vi "writeToXML.vi"(8 "error in (no error)":errorcluster, 10 "classLabel":string, 11 "StartUp in":refnum<class "StartUp.lvclass">) -> (0 "error out":errorcluster, 2 "XML out":string, 3 "StartUp out":refnum<class "StartUp.lvclass">)   [LabVIEW 2022 SP3, in "TCSDataDefinitions.lvlib" / "TCSCommand.lvlib" / "StartUp.lvclass"]
uses:
  StartUp.lvclass
  TCSTcsCommand/TCSTcsCommand.lvclass
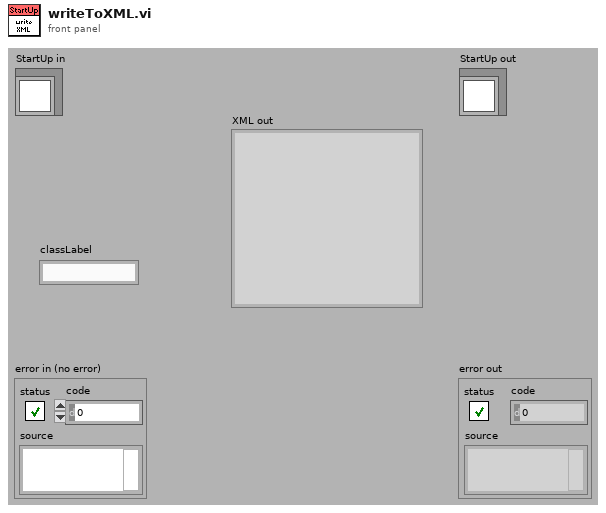
[diagram p1: front panel]
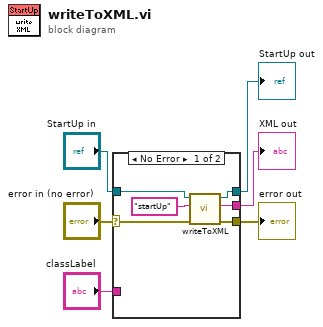
[diagram p0: block diagram]
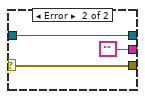
[diagram p2: hidden frame]
diagram:
  n1 = case shown="No Error" "error in (no error)" {
    selector: "error in (no error)" -> [w8 w15]
    tunnel: [w7 w15] -> w5
    tunnel: [w10 w14] -> w3
    tunnel: "StartUp in" -> [w11 w14]
    tunnel: [w9 ""] -> w2
    tunnel: "classLabel" -> [_ _]
    frame No Error {
      n2 = call-parent "writeToXML.vi"("error in (no error)"=w8, "ClassLabel"="startUp", "TCSTcsCommand in"=w11) -> ("error out"=w7:errorcluster, "XML out"=w9:string, "TCSTcsCommand out"=w10:refnum<class "StartUp.lvclass">)  [unwired: 6 in]
    }
    frame Error {
    }
  }
  "error out" <- w5
  "StartUp out" <- w3
  "XML out" <- w2
